vi "Limelight Control.vi"(10 "input cluster":T1={"DevStatus"={"status"=FALSE, "code"=0, "source"=""}, "Motors[]"=[], "Square Inputs"=FALSE, "Max Output"=1.0}) -> ()   [LabVIEW 2019]
uses:
  <vilib>/Rock Robotics/WPI/RobotDrive/WPI_RobotDriveDevRef.ctl
  <vilib>/Rock Robotics/WPI/MotorControl/WPI_MotorControlDeviceRef.ctl
  <vilib>/Rock Robotics/WPI/MotorControl/WPI_MotorControlType.ctl
  <vilib>/Rock Robotics/SystemInterfaces/DIO/FPGA_DIOPWMChannel.ctl
  <vilib>/Rock Robotics/WPI/PWM/WPI_PWMDeadband.ctl
  <vilib>/Rock Robotics/SystemInterfaces/DIO/FPGA_DIOChannel.ctl
  <vilib>/Rock Robotics/Network Tables/NT Read Number.vi
  <vilib>/addons/control/pid/pid.llb/PID (DBL).vi
  <vilib>/Rock Robotics/WPI/ThirdParty/Phoenix-LabVIEW/Motor Controller/Controls/CTRE_Phoenix_MotorControl_ControlMode.ctl
  <vilib>/addons/control/pid/NI_PID_pid.lvlib
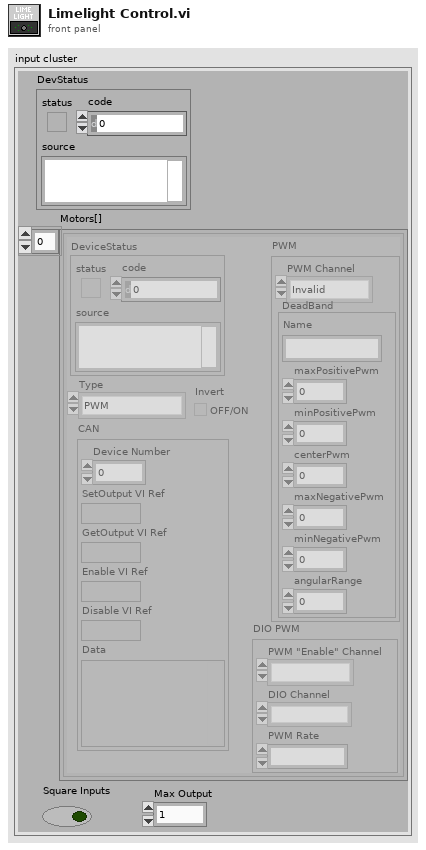
[diagram p1: front panel]
types:
  T1 = typedef "WPI_RobotDriveDevRef.ctl" = cluster{"DevStatus":errorcluster, "Motors[]":T2[], "Square Inputs":bool, "Max Output":dbl}
  T2 = typedef "WPI_MotorControlDeviceRef.ctl" = cluster{"DeviceStatus":errorcluster, "Type":T3, "PWM":cluster{"PWM Channel":T4, "DeadBand":T5}, "CAN":cluster{"Device Number":u8, "SetOutput VI Ref":variant, "GetOutput VI Ref":variant, "Enable VI Ref":variant, "Disable VI Ref":variant, "Data":variant}, "Invert":bool, "DIO PWM":cluster{"PWM \"Enable\" Channel":T4, "DIOChannel":T6, "PWM Rate":dbl}}
  T3 = typedef "WPI_MotorControlType.ctl" = enum16{"PWM", "CAN", "DIO PWM"}
  T4 = typedef "FPGA_DIOPWMChannel.ctl" = enum8{"PWM 0", "PWM 1", "PWM 2", "PWM 3", "PWM 4", "PWM 5", "PWM 6", "PWM 7", "PWM 8", "PWM 9", "PWM MXP 0", "PWM MXP 1", "PWM MXP 2", "PWM MXP 3", "PWM MXP 4", "PWM MXP 5", "PWM MXP 6", "PWM MXP 7", "PWM MXP 8", "PWM MXP 9", "Invalid"}
  T5 = typedef "WPI_PWMDeadband.ctl" = cluster{"Name":string, "maxPositivePwm":i32, "minPositivePwm":i32, "centerPwm":i32, "maxNegativePwm":i32, "minNegativePwm":i32, "angularRange":u16}
  T6 = typedef "FPGA_DIOChannel.ctl" = enum8{"DIO 0", "DIO 1", "DIO 2", "DIO 3", "DIO 4", "DIO 5", "DIO 6", "DIO 7", "DIO 8", "DIO 9", "DIO MXP 0", "DIO MXP 1", "DIO MXP 2", "DIO MXP 3", "DIO MXP 4", "DIO MXP 5", "DIO MXP 6", "DIO MXP 7", "DIO MXP 8", "DIO MXP 9", "DIO MXP 10", "DIO MXP 11", "DIO MXP 12", "DIO MXP 13", "DIO MXP 14", "DIO MXP 15", "SPI Port CS1", "SPI Port CS2", "SPI Port CS3", "SPI Port MISO", "SPI Port MOSI", "Invalid"}
  T7 = cluster{"proportional gain (Kc)":dbl, "integral time (Ti, min)":dbl, "derivative time (Td, min)":dbl}
  T8 = typedef "CTRE_Phoenix_MotorControl_ControlMode.ctl" = u16
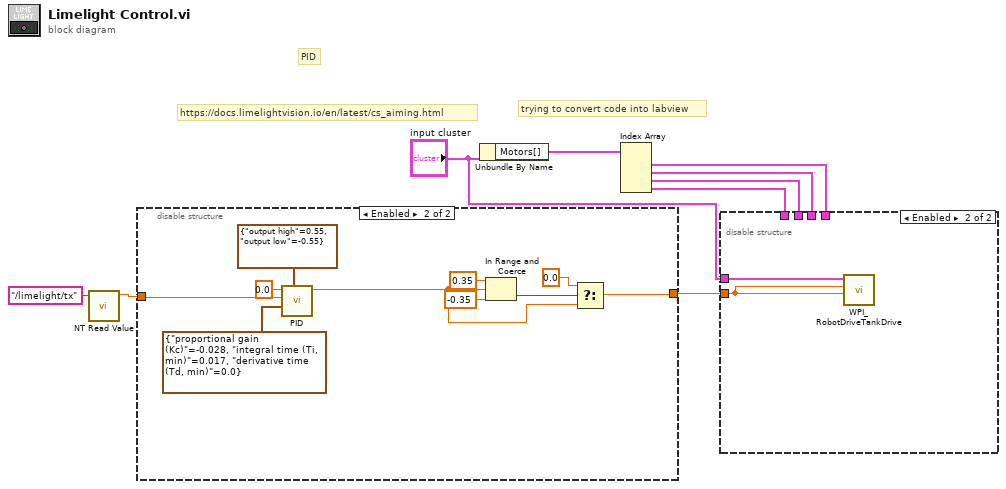
[diagram p0: block diagram]
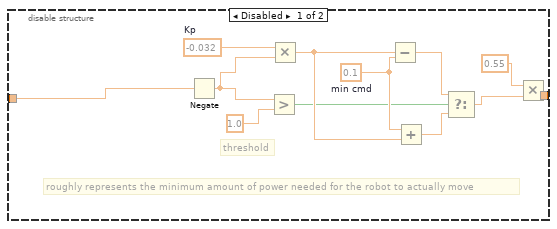
[diagram p2: hidden frame]
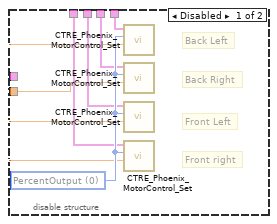
[diagram p3: hidden frame]
diagram:
  # "PID"
  # "trying to convert code into labview"
  # "https://docs.limelightvision.io/en/latest/cs_aiming.html"
  n1 = call-poly <vilib>:"NT Read Value.vi"("Name"="/limelight/tx") -> ("Numeric"=w1:dbl)  [unwired: 9 in, 1 out]
  n2 = disable-structure shown="Enabled" {
    disable-tunnel: [w21 w23] -> w4
    disable-tunnel: w1 -> [w13 w31]
    frame Disabled {
      w18 = 0.1  # min cmd
      w16 = -0.032  # Kp
      # "roughly represents the minimum amount of power needed for the robot to actually move"
      # "threshold"
      n3 = Negate(x=w13) -> (-x=w12:dbl)
      n4 = Greater?(x=w12, y=1.0) -> (0:w15:bool)
      n5 = Multiply(x=w16, y=w12) -> (x*y=w19:dbl)
      n6 = Subtract(x=w19, y=w18) -> (x-y=w17:dbl)
      n7 = Add(x=w18, y=w19) -> (x+y=w20:dbl)
      n8 = Select(t=w17, s=w15, f=w20) -> (s? t:f=w10:dbl)
      n9 = Multiply(x=0.55, y=w10) -> (x*y=w21:dbl)
    }
    frame Enabled {
      n10 = call-poly <vilib>:"PID.vi"("output range"=cluster{"output high":dbl, "output low":dbl} {"output high"=0.55, "output low"=-0.55}, "PID gains"=T7 {"proportional gain (Kc)"=-0.028, "integral time (Ti, min)"=0.017, "derivative time (Td, min)"=0.0}, "process variable"=w31, "setpoint"=0.0) -> ("output"=w24:dbl)  [unwired: 6 in, 1 out]
      n11 = In Range and Coerce(upper limit=0.35, x=w24, lower limit=-0.35) -> (In Range?=w25:bool)  [unwired: 1 out]
      n12 = Select(t=0.0, s=w25, f=w24) -> (s? t:f=w23:dbl)
    }
  }
  n13 = Unbundle By Name("input cluster") -> ("Motors[]"=w5:T2[])
  n14 = Index Array(array=w5) -> (element #1=w6:T2, element #2=w7:T2, element #3=w8:T2, element #4=w9:T2)  [unwired: 4 in]
  n15 = disable-structure shown="Enabled" {
    disable-tunnel: w9 -> [w36 _]
    disable-tunnel: w8 -> [w35 _]
    disable-tunnel: w7 -> [w34 _]
    disable-tunnel: w6 -> [w33 _]
    disable-tunnel: w4 -> [w32 w39]
    disable-tunnel: "input cluster" -> [_ w38]
    frame Disabled {
      w37 = T8 0 items=["PercentOutput"=0, "Position"=1, "Velocity"=2, "Current"=3, "Follower"=5, "MotionProfile"=6, "MotionMagic"=7, "MotionProfileArc"=10, "Disabled"=15] ("Control Mode")
      # "Front right"
      # "Front Left"
      # "Back Right"
      # "Back Left"
      n16 = call <vilib>:"CTRE_Phoenix_MotorControl_Set.vi"("Output"=w32, "Control Mode"=w37, "PhoenixMotorControlDevRef"=w33) -> ()  [unwired: 7 in, 2 out]
      n17 = call <vilib>:"CTRE_Phoenix_MotorControl_Set.vi"("Output"=w32, "Control Mode"=w37, "PhoenixMotorControlDevRef"=w34) -> ()  [unwired: 7 in, 2 out]
      n18 = call <vilib>:"CTRE_Phoenix_MotorControl_Set.vi"("Output"=w32, "Control Mode"=w37, "PhoenixMotorControlDevRef"=w35) -> ()  [unwired: 7 in, 2 out]
      n19 = call <vilib>:"CTRE_Phoenix_MotorControl_Set.vi"("Output"=w32, "Control Mode"=w37, "PhoenixMotorControlDevRef"=w36) -> ()  [unwired: 7 in, 2 out]
    }
    frame Enabled {
      n20 = call <vilib>:"WPI_RobotDriveTankDrive.vi"("Right axis value"=w39, "Left axis value"=w39, "RobotDriveDevRef"=w38) -> ()  [unwired: 6 in, 3 out]
    }
  }
